vi "test.compress.buffer.vi"() -> (3 "All Passed":bool)   [LabVIEW 2020]
uses:
  compress.buffer.test.case.ctl
panel:
  out "Passed 9":bool
  in  "Test Case #9 - Remove Long Unaligned Buffer with 4 byte unaligned spill":T1={"buffer"=[4822678189205111, 1234605616436508552, 11072869122414935842, 8627565158402756932, 1311767949471645696, 0, 0, 0, 0], "buffer.length"=34, "start.idx"=30, "exp.buffer.length"=4, "exp.buffer"=[1244139411608698880, 0, 0, 0, 0, 0, 0, 0, 0]} {"exp.buffer" format="%016x"; "buffer" format="%016x"}
  out "Passed 8":bool
  in  "Test Case #8 - Remove Long Unaligned Buffer with 2 byte unaligned spill":T1={"buffer"=[4822678189205111, 1234605616436508552, 11072869122414935842, 8627565158402756932, 1311767949471645696, 0, 0, 0, 0], "buffer.length"=33, "start.idx"=31, "exp.buffer.length"=2, "exp.buffer"=[4904982944159891456, 0, 0, 0, 0, 0, 0, 0, 0]} {"exp.buffer" format="%016x"; "buffer" format="%016x"}
  out "Passed 7":bool
  in  "Test Case #7 - Remove Long Unaligned Buffer with 2 byte spill":T1={"buffer"=[4822678189205111, 1234605616436508552, 11072869122414935842, 8627565158402756932, 1311767949471645696, 0, 0, 0, 0], "buffer.length"=35, "start.idx"=34, "exp.buffer.length"=1, "exp.buffer"=[6196953087261802496, 0, 0, 0, 0, 0, 0, 0, 0]} {"exp.buffer" format="%016x"; "buffer" format="%016x"}
  out "Passed 6":bool
  in  "Test Case #6 - Remove Long Unaligned Buffer with no spill":T1={"buffer"=[4822678189205111, 1234605616436508552, 11072869122414935842, 8627565158402756932, 1311768467452592128, 0, 0, 0, 0], "buffer.length"=38, "start.idx"=33, "exp.buffer.length"=5, "exp.buffer"=[3771334341091655680, 0, 0, 0, 0, 0, 0, 0, 0]} {"exp.buffer" format="%016x"; "buffer" format="%016x"}
  out "Passed 5":bool
  in  "Test Case #5 - Remove Long Aligned Buffer with 6 extra bytes":T1={"buffer"=[4822678189205111, 43707, 0, 0, 0, 0, 0, 0, 0], "buffer.length"=10, "start.idx"=0, "exp.buffer.length"=2, "exp.buffer"=[12302426807092641792, 0, 0, 0, 0, 0, 0, 0, 0]} {"exp.buffer" format="%016x"; "buffer" format="%016x"}
  out "Passed 4":bool
  in  "Test Case #4 - Remove Long Aligned Buffer with 2 extra bytes":T1={"buffer"=[4822678189205111, 1234605616436508552, 11072869122414935842, 8627565158402756932, 1297036692682702848, 0, 0, 0, 0], "buffer.length"=10, "start.idx"=0, "exp.buffer.length"=1, "exp.buffer"=[1297036692682702848, 0, 0, 0, 0, 0, 0, 0, 0]} {"exp.buffer" format="%016x"; "buffer" format="%016x"}
  out "Passed 3":bool
  in  "Test Case #3 - Remove 6 bytes from 8 byte buffer (Time Message)":T1={"buffer"=[4822678189205111, 12278557582179740347, 0, 0, 0, 0, 0, 0, 0], "buffer.length"=8, "start.idx"=6, "exp.buffer.length"=2, "exp.buffer"=[7383370114097217536, 0, 0, 0, 0, 0, 0, 0, 0]} {"exp.buffer" format="%016x"; "buffer" format="%016x"}
  out "Passed 2":bool
  in  "Test Case #2 - Remove 8 bytes from 10 byte buffer (Seq Unit Hdr unaligned)":T1={"buffer"=[4822678189205111, 12302426807092641792, 0, 0, 0, 0, 0, 0, 0], "buffer.length"=10, "start.idx"=8, "exp.buffer.length"=2, "exp.buffer"=[12302426807092641792, 0, 0, 0, 0, 0, 0, 0, 0]} {"exp.buffer" format="%016x"; "buffer" format="%016x"}
  in  "Test Case #1 - Remove 8 bytes from 8 byte buffer":T1={"buffer"=[4822678189205111, 0, 0, 0, 0, 0, 0, 0, 0], "buffer.length"=8, "start.idx"=8, "exp.buffer.length"=0, "exp.buffer"=[0, 0, 0, 0, 0, 0, 0, 0, 0]} {"exp.buffer" format="%016x"; "buffer" format="%016x"}
  in  "Test #":i32=1
  in  "Override":bool
  out "Passed 1":bool=TRUE
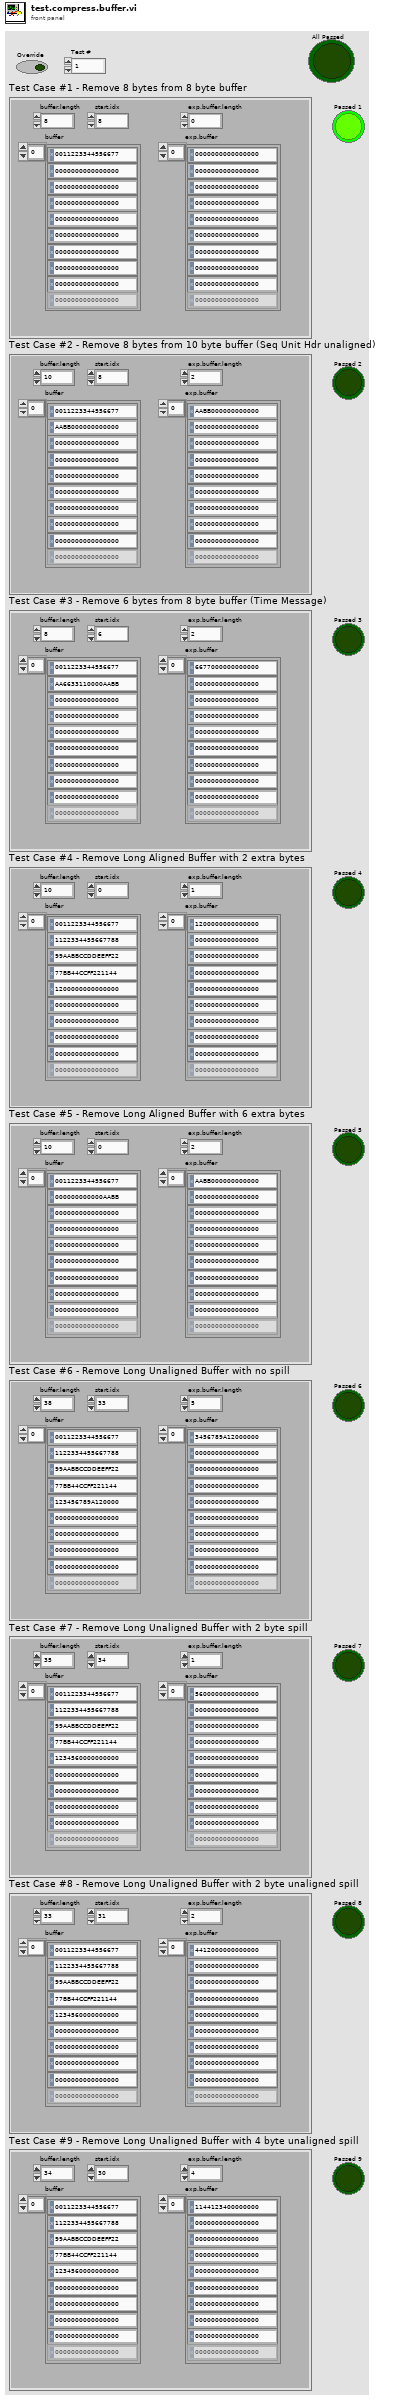
[diagram p1: front panel]
types:
  T1 = typedef "compress.buffer.test.case.ctl" = cluster{"buffer":u64[], "buffer.length":u8, "start.idx":u8, "exp.buffer.length":u8, "exp.buffer":u64[]}
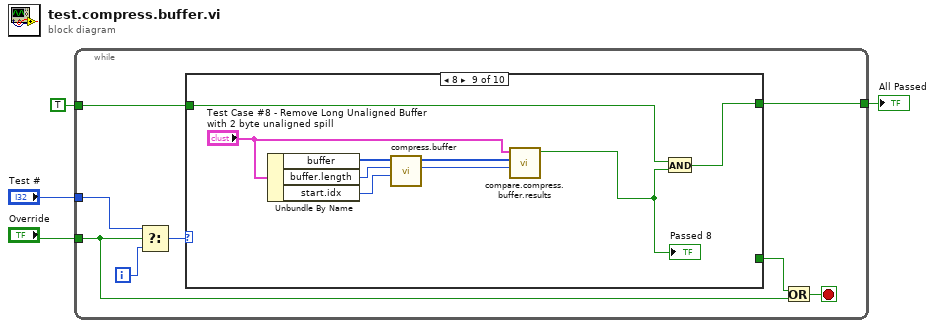
[diagram p0: block diagram]
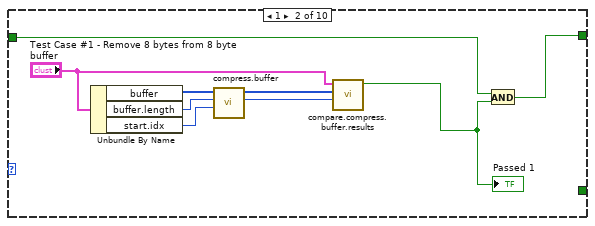
[diagram p3: hidden frame]
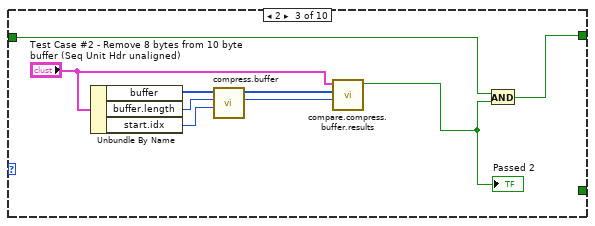
[diagram p4: hidden frame]
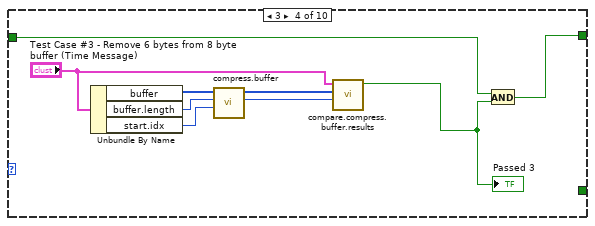
[diagram p5: hidden frame]
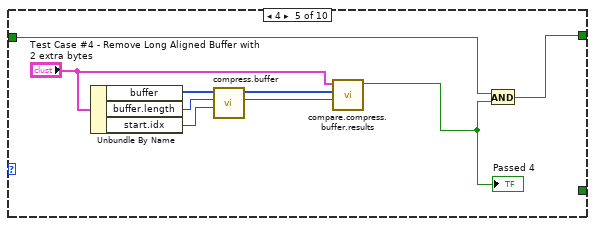
[diagram p6: hidden frame]
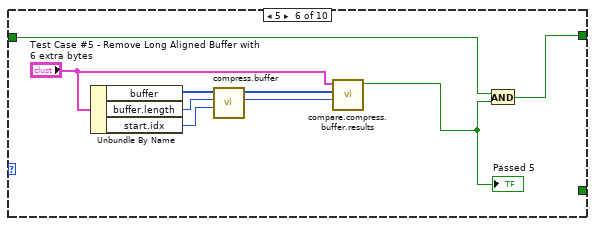
[diagram p7: hidden frame]
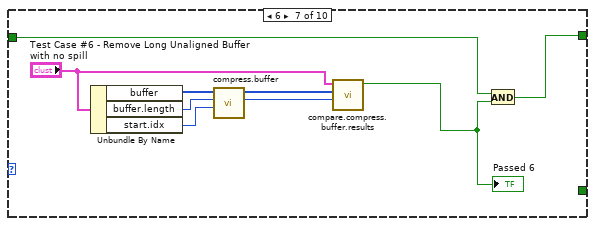
[diagram p8: hidden frame]
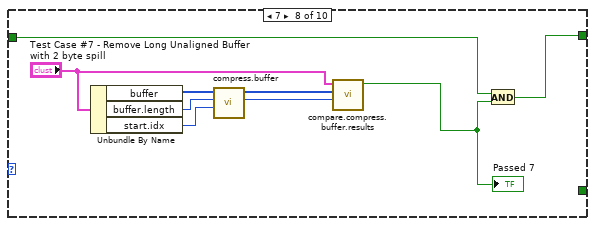
[diagram p9: hidden frame]
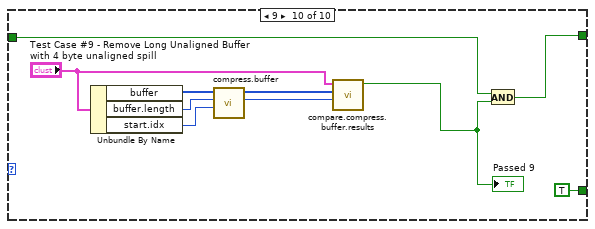
[diagram p10: hidden frame]
diagram:
  n1 = while {
    tunnel: TRUE -> [w11]
    tunnel: [w10] -> w1
    tunnel: "Test #" -> [w9]
    tunnel: "Override" -> [w5]
    i -> [w8]
    stop <- w6 stop-if-true
    n2 = Select(t=w9, s=w5, f=w8) -> (s? t:f=w7:i32)
    n3 = case shown="8" w7 {
      tunnel: [_ _ _ _ _ _ _ _ _ TRUE] -> w12
      tunnel: w11 -> [w13 w21 w30 w39 w48 w57 w66 w75 w84 w94]
      tunnel: [w13 w22 w31 w40 w49 w58 w67 w76 w85 w95] -> w10
      frame 0, Default {
      }
      frame 1 {
        n4 = Unbundle By Name("Test Case #1 - Remove 8 bytes from 8 byte buffer") -> ("buffer"=w20:u64[], "buffer.length"=w19:u8, "start.idx"=w18:u8)
        n5 = call "compress.buffer.vi"("start.idx"=w18, "buffer.length"=w19, "buffer"=w20) -> ("buffer.length.out"=w15:u8, "buffer.out"=w16:u64[])  [unwired: 7 in]
        n6 = call "compare.compress.buffer.results.vi"("buffer.length.out"=w15, "buffer.out"=w16, "Test Case"="Test Case #1 - Remove 8 bytes from 8 byte buffer") -> ("Passed?"=w14:bool)  [unwired: 6 in, 2 out]
        "Passed 1" <- w14
        n7 = And(x=w21, y=w14) -> (x .and. y?=w22:bool)
      }
      frame 2 {
        n8 = Unbundle By Name("Test Case #2 - Remove 8 bytes from 10 byte buffer (Seq Unit Hdr unaligned)") -> ("buffer"=w29:u64[], "buffer.length"=w28:u8, "start.idx"=w27:u8)
        n9 = call "compress.buffer.vi"("start.idx"=w27, "buffer.length"=w28, "buffer"=w29) -> ("buffer.length.out"=w24:u8, "buffer.out"=w25:u64[])  [unwired: 7 in]
        n10 = call "compare.compress.buffer.results.vi"("buffer.length.out"=w24, "buffer.out"=w25, "Test Case"="Test Case #2 - Remove 8 bytes from 10 byte buffer (Seq Unit Hdr unaligned)") -> ("Passed?"=w23:bool)  [unwired: 6 in, 2 out]
        "Passed 2" <- w23
        n11 = And(x=w30, y=w23) -> (x .and. y?=w31:bool)
      }
      frame 3 {
        n12 = Unbundle By Name("Test Case #3 - Remove 6 bytes from 8 byte buffer (Time Message)") -> ("buffer"=w38:u64[], "buffer.length"=w37:u8, "start.idx"=w36:u8)
        n13 = call "compress.buffer.vi"("start.idx"=w36, "buffer.length"=w37, "buffer"=w38) -> ("buffer.length.out"=w33:u8, "buffer.out"=w34:u64[])  [unwired: 7 in]
        n14 = call "compare.compress.buffer.results.vi"("buffer.length.out"=w33, "buffer.out"=w34, "Test Case"="Test Case #3 - Remove 6 bytes from 8 byte buffer (Time Message)") -> ("Passed?"=w32:bool)  [unwired: 6 in, 2 out]
        "Passed 3" <- w32
        n15 = And(x=w39, y=w32) -> (x .and. y?=w40:bool)
      }
      frame 4 {
        n16 = Unbundle By Name("Test Case #4 - Remove Long Aligned Buffer with 2 extra bytes") -> ("buffer"=w47:u64[], "buffer.length"=w46:u8, "start.idx"=w45:u8)
        n17 = call "compress.buffer.vi"("start.idx"=w45, "buffer.length"=w46, "buffer"=w47) -> ("buffer.length.out"=w42:u8, "buffer.out"=w43:u64[])  [unwired: 7 in]
        n18 = call "compare.compress.buffer.results.vi"("buffer.length.out"=w42, "buffer.out"=w43, "Test Case"="Test Case #4 - Remove Long Aligned Buffer with 2 extra bytes") -> ("Passed?"=w41:bool)  [unwired: 6 in, 2 out]
        "Passed 4" <- w41
        n19 = And(x=w48, y=w41) -> (x .and. y?=w49:bool)
      }
      frame 5 {
        n20 = Unbundle By Name("Test Case #5 - Remove Long Aligned Buffer with 6 extra bytes") -> ("buffer"=w56:u64[], "buffer.length"=w55:u8, "start.idx"=w54:u8)
        n21 = call "compress.buffer.vi"("start.idx"=w54, "buffer.length"=w55, "buffer"=w56) -> ("buffer.length.out"=w51:u8, "buffer.out"=w52:u64[])  [unwired: 7 in]
        n22 = call "compare.compress.buffer.results.vi"("buffer.length.out"=w51, "buffer.out"=w52, "Test Case"="Test Case #5 - Remove Long Aligned Buffer with 6 extra bytes") -> ("Passed?"=w50:bool)  [unwired: 6 in, 2 out]
        "Passed 5" <- w50
        n23 = And(x=w57, y=w50) -> (x .and. y?=w58:bool)
      }
      frame 6 {
        n24 = Unbundle By Name("Test Case #6 - Remove Long Unaligned Buffer with no spill") -> ("buffer"=w65:u64[], "buffer.length"=w64:u8, "start.idx"=w63:u8)
        n25 = call "compress.buffer.vi"("start.idx"=w63, "buffer.length"=w64, "buffer"=w65) -> ("buffer.length.out"=w60:u8, "buffer.out"=w61:u64[])  [unwired: 7 in]
        n26 = call "compare.compress.buffer.results.vi"("buffer.length.out"=w60, "buffer.out"=w61, "Test Case"="Test Case #6 - Remove Long Unaligned Buffer with no spill") -> ("Passed?"=w59:bool)  [unwired: 6 in, 2 out]
        "Passed 6" <- w59
        n27 = And(x=w66, y=w59) -> (x .and. y?=w67:bool)
      }
      frame 7 {
        n28 = Unbundle By Name("Test Case #7 - Remove Long Unaligned Buffer with 2 byte spill") -> ("buffer"=w74:u64[], "buffer.length"=w73:u8, "start.idx"=w72:u8)
        n29 = call "compress.buffer.vi"("start.idx"=w72, "buffer.length"=w73, "buffer"=w74) -> ("buffer.length.out"=w69:u8, "buffer.out"=w70:u64[])  [unwired: 7 in]
        n30 = call "compare.compress.buffer.results.vi"("buffer.length.out"=w69, "buffer.out"=w70, "Test Case"="Test Case #7 - Remove Long Unaligned Buffer with 2 byte spill") -> ("Passed?"=w68:bool)  [unwired: 6 in, 2 out]
        "Passed 7" <- w68
        n31 = And(x=w75, y=w68) -> (x .and. y?=w76:bool)
      }
      frame 8 {
        n32 = Unbundle By Name("Test Case #8 - Remove Long Unaligned Buffer with 2 byte unaligned spill") -> ("buffer"=w83:u64[], "buffer.length"=w82:u8, "start.idx"=w81:u8)
        n33 = call "compress.buffer.vi"("start.idx"=w81, "buffer.length"=w82, "buffer"=w83) -> ("buffer.length.out"=w78:u8, "buffer.out"=w79:u64[])  [unwired: 7 in]
        n34 = call "compare.compress.buffer.results.vi"("buffer.length.out"=w78, "buffer.out"=w79, "Test Case"="Test Case #8 - Remove Long Unaligned Buffer with 2 byte unaligned spill") -> ("Passed?"=w77:bool)  [unwired: 6 in, 2 out]
        "Passed 8" <- w77
        n35 = And(x=w84, y=w77) -> (x .and. y?=w85:bool)
      }
      frame 9 {
        n36 = Unbundle By Name("Test Case #9 - Remove Long Unaligned Buffer with 4 byte unaligned spill") -> ("buffer"=w93:u64[], "buffer.length"=w92:u8, "start.idx"=w91:u8)
        n37 = call "compress.buffer.vi"("start.idx"=w91, "buffer.length"=w92, "buffer"=w93) -> ("buffer.length.out"=w88:u8, "buffer.out"=w89:u64[])  [unwired: 7 in]
        n38 = call "compare.compress.buffer.results.vi"("buffer.length.out"=w88, "buffer.out"=w89, "Test Case"="Test Case #9 - Remove Long Unaligned Buffer with 4 byte unaligned spill") -> ("Passed?"=w87:bool)  [unwired: 6 in, 2 out]
        "Passed 9" <- w87
        n39 = And(x=w94, y=w87) -> (x .and. y?=w95:bool)
      }
    }
    n40 = Or(x=w12, y=w5) -> (x .or. y?=w6:bool)
  }
  "All Passed" <- w1
